vi "SPD.HV_Grid Max Search.vi"(6 "HV_start":dbl, 7 "Continue":refnum<vi>, 8 "Error In":errorcluster, 9 "min step":dbl=32.0 format="%#_13g", 10 "HV_GridParams":T1, 11 "SPD.Stand Ctrl in":T2 {"spdDeviceSession"."hidSPD.Sturtup Values"."HV_bias" format="%#_6p, V"; "spdDeviceSession"."hidSPD.Sturtup Values"."TSet" format="%#_6p, DegC"; "spdDeviceSession"."hidSPD.Controller"."HV_bias" format="%#_6p, V"; "spdDeviceSession"."hidSPD.Controller"."TSet" format="%#_6p, DegC"}) -> (0 "Error Out":errorcluster, 1 "pass":bool, 2 "HV_bias max":dbl, 3 "SPD.Stand Ctrl out":T2 {"spdDeviceSession"."hidSPD.Sturtup Values"."HV_bias" format="%#_6p, V"; "spdDeviceSession"."hidSPD.Sturtup Values"."TSet" format="%#_6p, DegC"; "spdDeviceSession"."hidSPD.Controller"."HV_bias" format="%#_6p, V"; "spdDeviceSession"."hidSPD.Controller"."TSet" format="%#_6p, DegC"})   [LabVIEW 2018]
uses:
  typedefs/SPD.Stand Ctrl.ctl
  Instruments/SPD HID Interface/hidSPDLibForLabView/LibVIs/hidSPD Controls/hidSPD Device Session.ctl
  Instruments/SPD HID Interface/hidSPDLibForLabView/LibVIs/hidSPD Controls/hidSPD Controller.ctl
  Instruments/SPD HID Interface/hidSPDLibForLabView/LibVIs/hidSPD Controls/hidSPD SPD Type.ctl
  Instruments/KC705 DevBoard/typedefs/DevB.Session.ctl
  Instruments/KeySight 53230A/typedefs/FreqC.Session.ctl
  Instruments/KeySight 8164B/KeySight 8164B LAN InstrLib/typedefs/KeySight 8164B control.ctl
  Instruments/LeCroy SDA830/typedefs/LeCroy.Session.ctl
  typedefs/SPD.Events.ctl
  ConfigFile/SPD.Config File ctrl.ctl
  <vilib>/Utility/config.llb/Config Data RefNum.ctl
  typedefs/SPD.Meas Result.ctl
  typedefs/SPD.Queues.ctl
  typedefs/SPD.Stand state.ctl
  typedefs/SPD.HV_Grid Test Params.ctl
  SubVIs/comparison mode.ctl
  SubVIs/Min_Max.ctl
  Instruments/KeySight 8164B/KeySight 8164B LAN InstrLib.lvlib
  <vilib>/Utility/config.llb/NI_LVConfig.lvlib
  Instruments/SPD HID Interface/hidSPDLibForLabView/hidSPDLibForLabView.lvlib
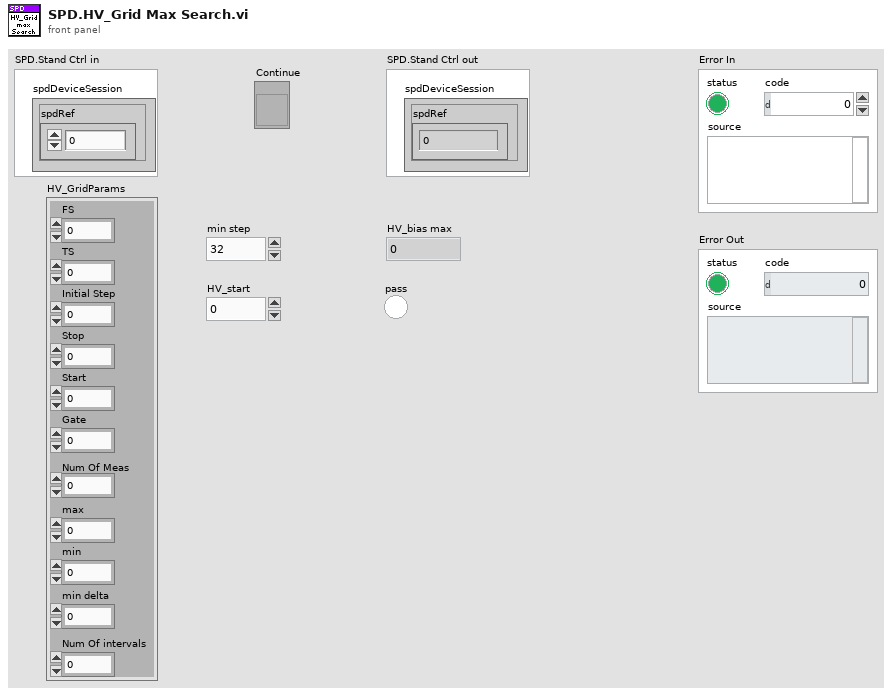
[diagram p1: front panel]
types:
  T1 = typedef "SPD.HV_Grid Test Params.ctl" = cluster{"FS":i32, "TS":i32, "Initial Step":dbl, "Stop":dbl, "Start":dbl, "Gate":dbl, "Num Of Meas":i32, "max":dbl, "min":dbl, "min delta":dbl, "Num Of intervals":i32}
  T2 = typedef "SPD.Stand Ctrl.ctl" = cluster{"spdDeviceSession":T3, "DevBSession":T6, "FreqCSession":T7, "8164BSession":T8, "LeCroySession":T9, "Events":T10, "configFile":T11, "SPD.Result":T13, "SPD.Queues":T14, "Console":refnum<vi>}
  T3 = typedef "hidSPDLibForLabView.lvlib/hidSPD Device Session.ctl" = cluster{"spdRef":u64, "connected":bool, "spdName":string, "hidSPD.Controller":T4, "hidSPD.Sturtup Values":T4, "SPD Type":T5}
  T4 = typedef "hidSPDLibForLabView.lvlib/hidSPD Controller.ctl" = cluster{"TSet":sgl, "HV_bias":sgl, "DDS_stb_code":u16}
  T5 = typedef "hidSPDLibForLabView.lvlib/hidSPD SPD Type.ctl" = enum16{"Free Run", "Gate"}
  T6 = typedef "DevB.Session.ctl" = cluster{"DevBRef":refnum<visa-resource-name>, "connected":bool}
  T7 = typedef "FreqC.Session.ctl" = cluster{"FreqCRef":refnum<visa-resource-name>, "timeout":dbl, "Gate":dbl, "connected":bool}
  T8 = typedef "KeySight 8164B LAN InstrLib.lvlib/KeySight 8164B control.ctl" = cluster{"Connection ID":refnum<k5>, "Connected":bool, "Info":string, "Slots Info":string[]}
  T9 = typedef "LeCroy.Session.ctl" = cluster{"LeCroySession":refnum<visa-resource-name>, "connected":bool}
  T10 = typedef "SPD.Events.ctl" = cluster{"DCRTest":refnum<user-event>, "Stop":refnum<user-event>}
  T11 = typedef "SPD.Config File ctrl.ctl" = cluster{"configFile ref":T12, "configFile path":path, "equipmentFile ref":T12}
  T12 = typedef "NI_LVConfig.lvlib/Config Data RefNum.ctl" = refnum<k1>
  T13 = typedef "SPD.Meas Result.ctl" = cluster{"HV_Bias":dbl[][][], "Stb_code":dbl[], "Temprature":dbl[], "Data":dbl[][][][], "DateTime":string}
  T14 = typedef "SPD.Queues.ctl" = cluster{"state queue":refnum<queue>}
  T15 = typedef "Min_Max.ctl" = cluster{"min":dbl, "max":dbl}
  T16 = typedef "comparison mode.ctl" = enum16{"in range", "bigger then min", "bigger then max", "less then min", "less then max"}
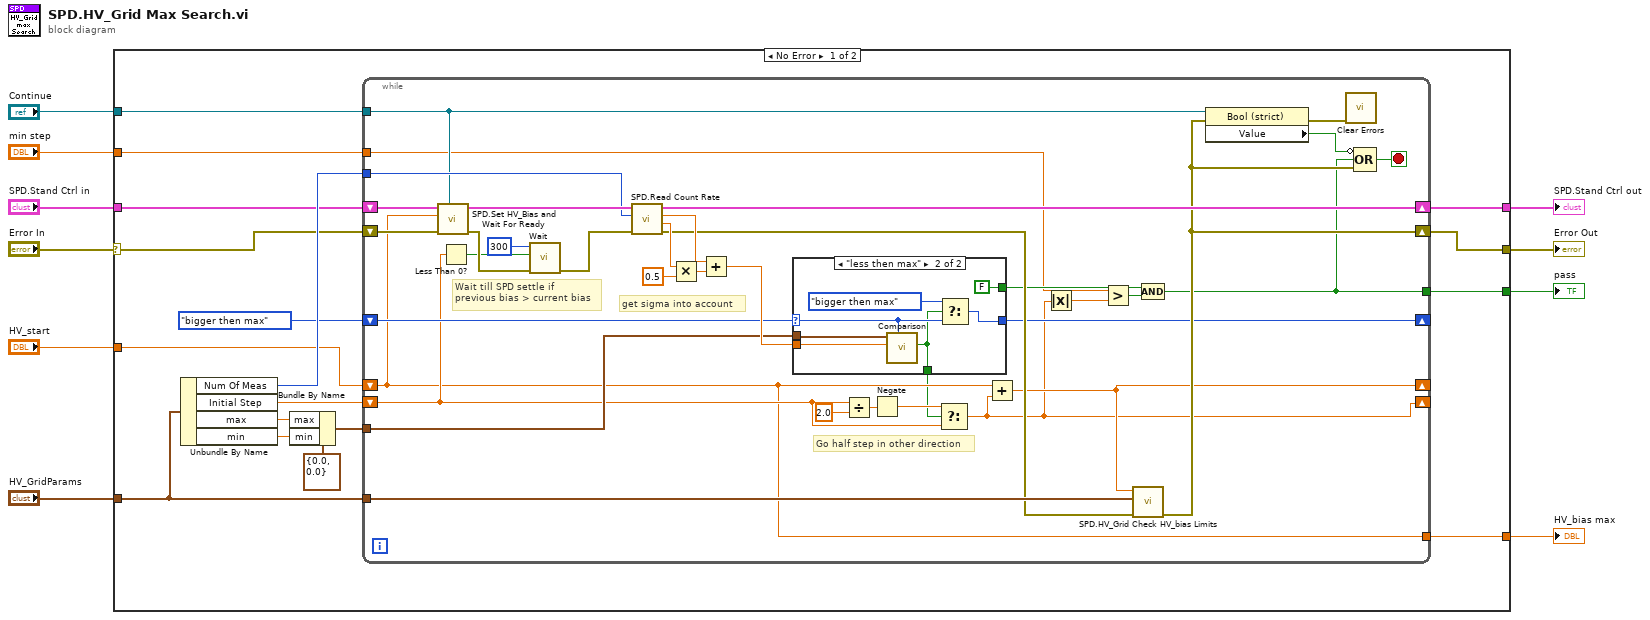
[diagram p0: block diagram]
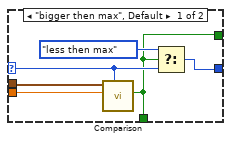
[diagram p2: hidden frame]
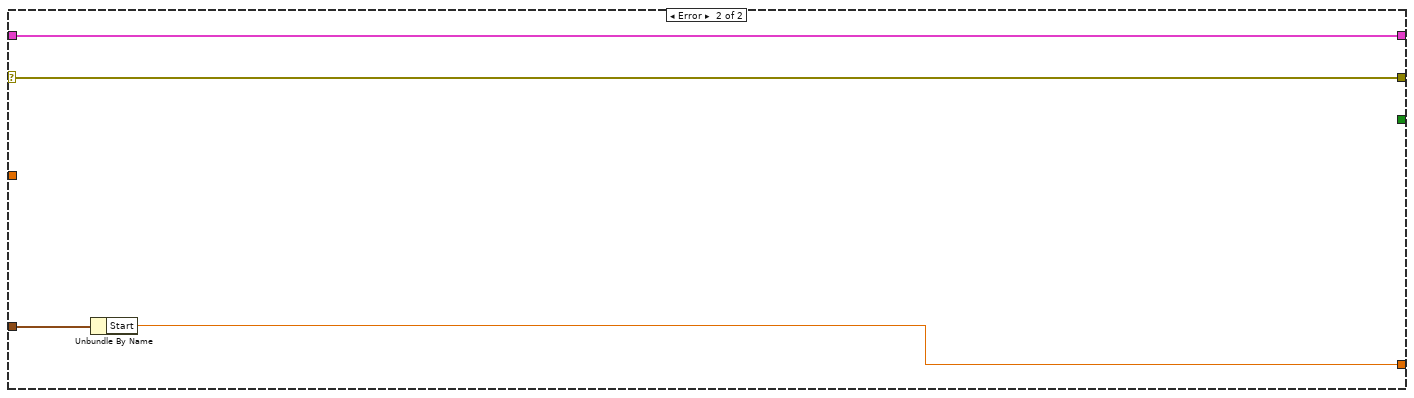
[diagram p3: hidden frame]
diagram:
  n1 = case shown="No Error" "Error In" {
    selector: "Error In" -> [w11 w81]
    tunnel: "Continue" -> [w27 _]
    tunnel: "SPD.Stand Ctrl in" -> [w25 w80]
    tunnel: [w24 w80] -> w8
    tunnel: [w23 w81] -> w7
    tunnel: "HV_GridParams" -> [w22 w79]
    tunnel: [w20 w78] -> w5
    tunnel: [w14 _] -> w4
    tunnel: "min step" -> [w13 _]
    tunnel: "HV_start" -> [w12 _]
    frame No Error {
      n2 = Unbundle By Name(w22) -> ("Num Of Meas"=w26:i32, "Initial Step"=w15:dbl, "max"=w18:dbl, "min"=w17:dbl)
      n3 = Bundle By Name(cluster=T15 {"min"=0.0, "max"=0.0} ("minMax"), "max"=w18, "min"=w17) -> (w16:T15)
      n4 = while {
        tunnel: w27 -> [w52]
        tunnel: w26 -> [w63]
        shift-right: [w57] -> w24
        shift-left: w25 -> [w58]
        shift-right: [w34] -> _
        shift-left: w12 -> [w40]
        shift-right: [w51] -> w23
        shift-left: w11 -> [w56]
        tunnel: w22 -> [w55]
        shift-right: [w30] -> _
        shift-left: w15 -> [w42]
        shift-right: [w39] -> _
        shift-left: comparison_mode."bigger then max" ("Comparison Mode") -> [w44]
        tunnel: [w40] -> w20
        tunnel: w16 -> [w43]
        tunnel: w13 -> [w31]
        tunnel: [w29] -> w14
        stop <- w54 stop-if-true
        # "Go half step in other direction"
        # "get sigma into account"
        # "Wait till SPD settle if \nprevious bias > current bias"
        n5 = call "SPD.Set HV_Bias and Wait For Ready.vi"("Continue"=w52, "Error In"=w56, "HV_Bias"=w40, "SPD.Stand Ctrl in"=w58) -> ("Error Out"=w46:errorcluster, "SPD.Stand Ctrl out"=w64:T2)  [unwired: 6 in]
        n6 = Less Than 0?(x=w42) -> (x < 0?=w45:bool)
        n7 = call "Wait.vi"("error in (no error)"=w46, "wait? (true)"=w45, "milliseconds to wait"=u32 300) -> ("error out"=w48:errorcluster)  [unwired: 8 in]
        n8 = call "SPD.Read Count Rate.vi"("Error In"=w48, "Num of Meas"=w63, "SPD.Stand Ctrl in"=w64) -> ("Error Out"=w41:errorcluster, "Count sigma"=w60:dbl, "Count"=w59:dbl, "SPD.Stand Ctrl out"=w57:T2)  [unwired: 5 in]
        n9 = Multiply(x=w60, y=0.5) -> (x*y=w62:dbl)
        n10 = Add(x=w59, y=w62) -> (x+y=w53:dbl)
        n11 = case shown="\"less then max\"" w44 {
          selector: w44 -> [w68 w75]
          tunnel: w53 -> [w70 w77]
          tunnel: w43 -> [w69 w76]
          tunnel: [w66 w73] -> w39
          tunnel: [w65 w72] -> w36
          tunnel: [w65 FALSE ("result")] -> w33
          frame "bigger then max", Default {
            n12 = call "Comparison.vi"("Comparison Mode"=w68, "value"=w70, "minMax"=w69) -> ("result"=w65:bool)  [unwired: 8 in]
            n13 = Select(t=comparison_mode."less then max", s=w65, f=w68) -> (s? t:f=w66:T16)
          }
          frame "less then max" {
            n14 = call "Comparison.vi"("Comparison Mode"=w75, "value"=w77, "minMax"=w76) -> ("result"=w72:bool)  [unwired: 8 in]
            n15 = Select(t=comparison_mode."bigger then max", s=w72, f=w75) -> (s? t:f=w73:T16)
          }
        }
        n16 = Divide(x=w42, y=2.0) -> (x/y=w37:dbl)
        n17 = Negate(x=w37) -> (-x=w38:dbl)
        n18 = Select(t=w38, s=w36, f=w42) -> (s? t:f=w30:dbl)
        n19 = Add(x=w40, y=w30) -> (x+y=w34:dbl)
        n20 = Absolute Value(x=w30) -> (abs(x)=w28:dbl)
        n21 = Greater?(x=w31, y=w28) -> (0:w32:bool)
        n22 = call "SPD.HV_Grid Check HV_bias Limits.vi"("Error In"=w41, "HV_GridParams"=w55, "Next HV_bias"=w34) -> ("Error Out"=w51:errorcluster)  [unwired: 8 in]
        n23 = Compound Arithmetic op=AND(w33, w32) -> (w29:bool)
        n24 = property class="Bool (strict)"(reference=w52, error in=w51) -> (error out=w49:errorcluster, "Value"=w50:bool)  [unwired: 1 out]
        n25 = call <vilib>:"Clear Errors.vi"("error in (no error)"=w49) -> ()  [unwired: 5 in, 2 out]
        n26 = Compound Arithmetic op=OR(invert w50, w29, w51) -> (w54:bool)
      }
    }
    frame Error {
      n27 = Unbundle By Name(w79) -> ("Start"=w78:dbl)
    }
  }
  "SPD.Stand Ctrl out" <- w8
  "Error Out" <- w7
  "HV_bias max" <- w5
  "pass" <- w4
